vi "Read Frame Rate.vi"(8 "error in (no error)":errorcluster, 11 "Stream in":refnum<class "Stream.lvclass">) -> (0 "error out":errorcluster, 2 "Frame Rate (FPS)":dbl, 3 "Stream":refnum<class "Stream.lvclass">)   [LabVIEW 2020, in "capture.lvlib" / "Stream.lvclass"]
doc: "Read Frame Rate."
uses:
  Stream.lvclass
  Stream.lvclass/Stream.ctl
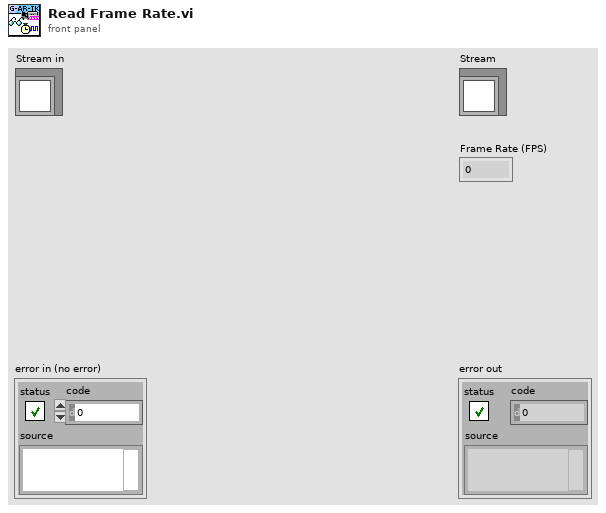
[diagram p1: front panel]
types:
  T1 = typedef "capture.lvlib/Stream.lvclass/Frames per Second.ctl" = cluster{"Numerator":u32, "Denominator":u32}
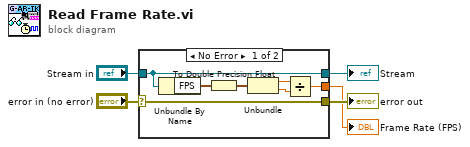
[diagram p0: block diagram]
diagram:
  n1 = case shown="No Error" "error in (no error)" {
    selector: "error in (no error)" -> [w12 w13]
    tunnel: [w12 w13] -> w4
    tunnel: [w11 w14] -> w2
    tunnel: "Stream in" -> [w11 w14]
    tunnel: [w7 _] -> w1
    frame No Error {
      n2 = Unbundle By Name(w11) -> ("FPS"=w10:T1)
      n3 = To Double Precision Float(number=w10) -> (double precision float=w9:cluster{"Numerator":dbl, "Denominator":dbl})
      n4 = Unbundle(w9) -> ("Numerator"=w8:dbl, "Denominator"=w6:dbl)
      n5 = Divide(x=w8, y=w6) -> (x/y=w7:dbl)
    }
    frame Error {
    }
  }
  "error out" <- w4
  "Stream" <- w2
  "Frame Rate (FPS)" <- w1
